vi "drone_havuz_uzaklık_uygulaması.vi"() -> ()   [LabVIEW 2018]
doc: "This example opens two VISA resources and configures one COM port to perform a write operation and the other COM port to perform a read operation. This VI will wait until the specified number of bytes is received at the port or until a termination character is read.\n\nThis example allows you perform diagnostic tests on your ports. You can use this example to perform a wrap-back test. Both serial ports must have the same basic configuration parameters. You can connect two of the ports using a null modem cable, which effectively connects one port's RX lines to the other port's TX lines. If you use a straight-through cable, one port's RX lines will be connected to the other port's RX lines, and you cannot communicate between the two ports."
uses:
  D:/Program Files (x86)/National Instruments/LabVIEW 2018/examples/Instrument IO/Serial/support/Serial - Settings.ctl
  <vilib>/Instr/_visa.llb/VISA Configure Serial Port (Instr).vi
panel:
  out "MESAFE GÖSTERGESİ":dbl(knob) scale=0.0..100.0
  out "Araç havuza çok uzak":bool
  out "Araç havuza uzak":bool
  out "Araç havuza yakın":bool
  in  "Termination Character":u8=10 format="%.0x"
  in  "End Write on Termination Character?":bool=TRUE
  in  "End Read on Termination Character?":bool=TRUE
  in  "Write String":string="*IDN?"
  in  "Serial Settings (read)":T1={"baud rate"=9600, "data bits"=8, "parity"=enum."None", "stop bits"=10, "flow control"=0} {"flow control" items=["None"=0, "XON/XOFF"=1, "RTS/CTS"=2, "DTR/DSR"=4]; "stop bits" items=["1.0"=10, "1.5"=15, "2.0"=20]; "data bits" min=5 max=8 step=1; "baud rate" items=["75"=75, "110"=110, "134"=134, "150"=150, "300"=300, "600"=600, "1200"=1200, "1800"=1800, "2400"=2400, "4800"=4800, "7200"=7200, "9600"=9600, "14400"=14400, "19200"=19200, "28800"=28800, "38400"=38400, "56000"=56000, "57600"=57600, "115200"=115200, "128000"=128000, "230400"=230400]}
  in  "Serial Settings (write)":T1={"baud rate"=9600, "data bits"=8, "parity"=enum."None", "stop bits"=10, "flow control"=0} {"flow control" items=["None"=0, "XON/XOFF"=1, "RTS/CTS"=2, "DTR/DSR"=4]; "stop bits" items=["1.0"=10, "1.5"=15, "2.0"=20]; "data bits" min=5 max=8 step=1; "baud rate" items=["75"=75, "110"=110, "134"=134, "150"=150, "300"=300, "600"=600, "1200"=1200, "1800"=1800, "2400"=2400, "4800"=4800, "7200"=7200, "9600"=9600, "14400"=14400, "19200"=19200, "28800"=28800, "38400"=38400, "56000"=56000, "57600"=57600, "115200"=115200, "128000"=128000, "230400"=230400]}
  out "bytes read":u32
  out "Read String":string
  in  "VISA Resource (read)":refnum<visa-resource-name>="COM2"
  out "bytes written":u32
  in  "VISA Resource (write)":refnum<visa-resource-name>="COM1"
  # "0xA is equivalent to a '\\n' character, which is a line feed."
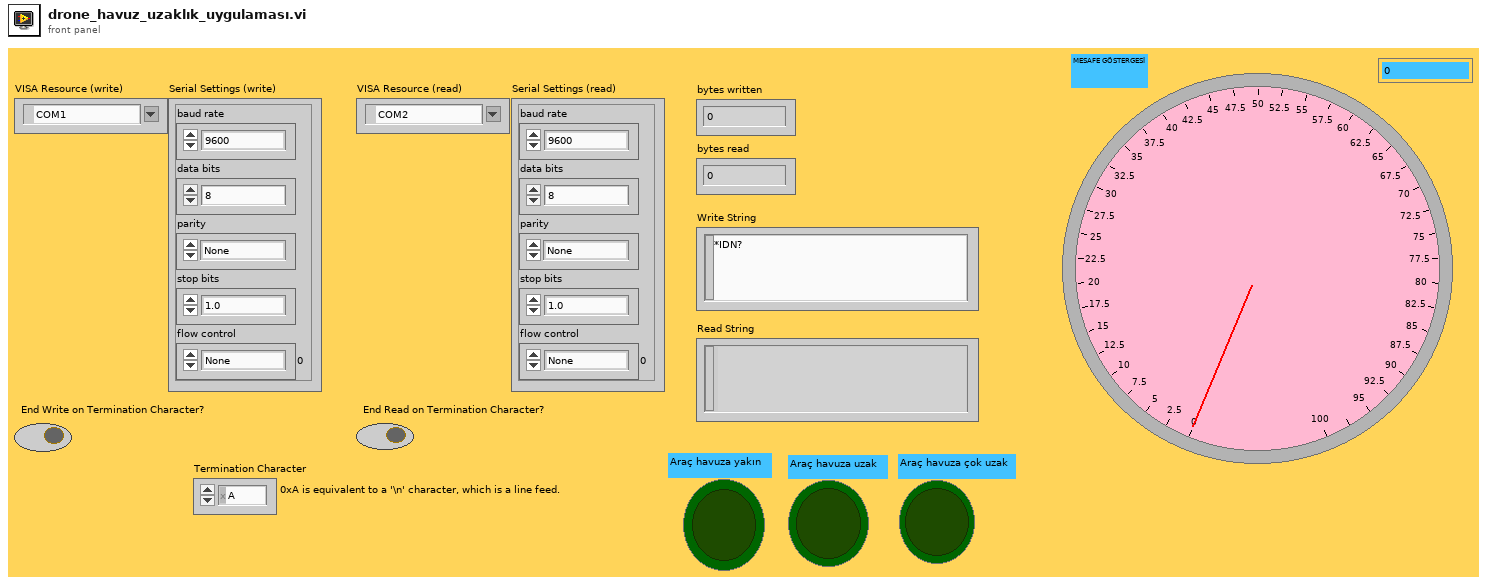
[diagram p1: front panel]
types:
  T1 = typedef "Serial - Settings.ctl" = cluster{"baud rate":u32, "data bits":u16, "parity":enum16{"None", "Odd", "Even", "Mark", "Space"}, "stop bits":u16, "flow control":u16}
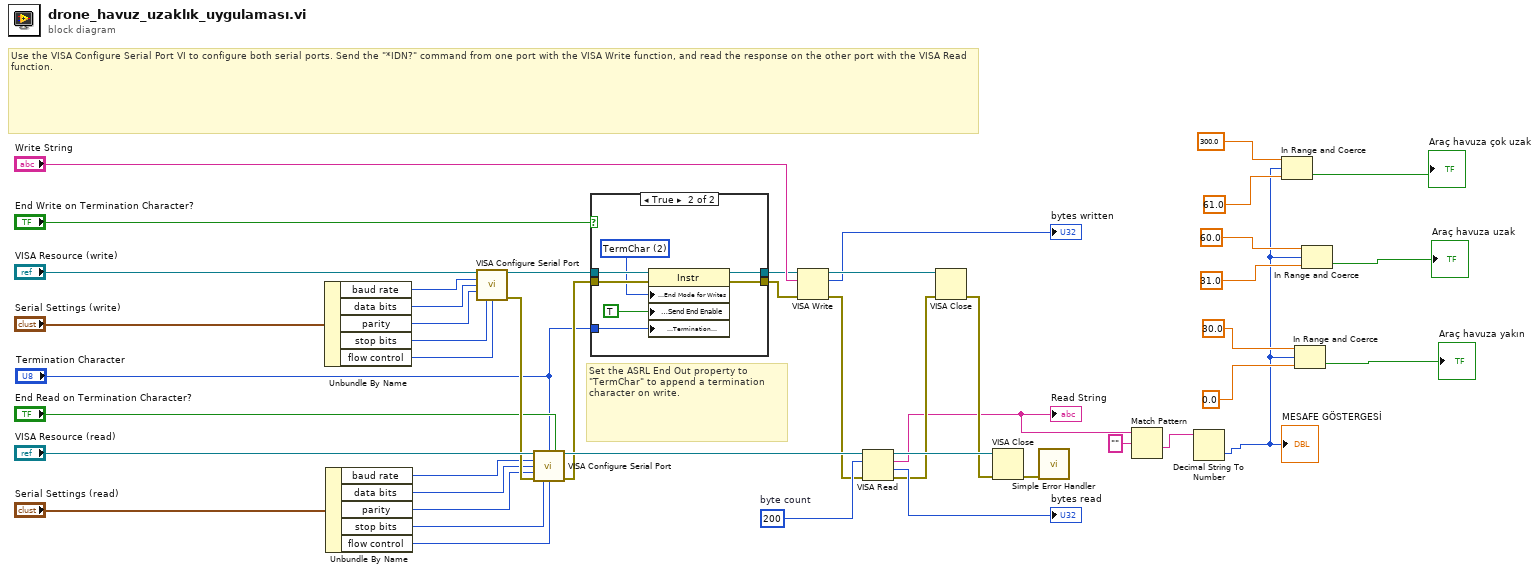
[diagram p0: block diagram]
diagram:
  w41 = u32 200  # byte count
  # "Set the ASRL End Out property to \"TermChar\" to append a termination character on write."
  # "Use the VISA Configure Serial Port VI to configure both serial ports. Send the \"*IDN?\" command from one port with the VISA Write function, and read the response on the other port with the VISA Read function."
  n1 = Unbundle By Name("Serial Settings (write)") -> ("baud rate"=w32:u32, "data bits"=w31:u16, "parity"=w30:enum16{"None", "Odd", "Even", "Mark", "Space"}, "stop bits"=w29:u16, "flow control"=w28:u16)
  n2 = Unbundle By Name("Serial Settings (read)") -> ("baud rate"=w26:u32, "data bits"=w25:u16, "parity"=w24:enum16{"None", "Odd", "Even", "Mark", "Space"}, "stop bits"=w23:u16, "flow control"=w22:u16)
  n3 = call-poly "VISA Configure Serial Port"("VISA resource name"="VISA Resource (write)", "baud rate (9600)"=w32, "data bits (8)"=w31, "parity (0:none)"=w30, "stop bits (10: 1 bit)"=w29, "flow control (0:none)"=w28) -> ("VISA resource name out"=w19:refnum<visa-resource-name>, "error out"=w38:errorcluster)  [unwired: 3 in, 5 out]
  n4 = call-poly "VISA Configure Serial Port"("VISA resource name"="VISA Resource (read)", "termination char\n(0xA = '\\n' = LF)"="Termination Character", "Enable Termination\nChar (T)"="End Read on Termination Character?", "baud rate (9600)"=w26, "data bits (8)"=w25, "parity (0:none)"=w24, "error in (no error)"=w38, "stop bits (10: 1 bit)"=w23, "flow control (0:none)"=w22) -> ("VISA resource name out"=w44:refnum<visa-resource-name>, "error out"=w17:errorcluster)  [unwired: 1 in, 4 out]
  n5 = case shown="True" "End Write on Termination Character?" {
    tunnel: w19 -> [w47 w55]
    tunnel: w17 -> [w48 w54]
    tunnel: [w47 w53] -> w18
    tunnel: [w48 w52] -> w16
    tunnel: "Termination Character" -> [_ w50]
    frame False {
    }
    frame True {
      w51 = u16 2 items=["None", "LastBit", "TermChar", "Break"] ("Serial Settings:Serial End Mode for Writes")
      n6 = property class="Instr"(reference=w55, error in=w54, "Serial Settings:End Mode for Writes"=w51, "Message Based Settings:Send End Enable"=TRUE, "Message Based Settings:Termination Character"=w50) -> (reference out=w53:refnum<visa-resource-name>, error out=w52:errorcluster)
    }
  }
  n7 = VISA Write(VISA resource name=w18, write buffer="Write String", error in (no error)=w16) -> (VISA resource name out=w45:refnum<visa-resource-name>, return count=→"bytes written":u32, error out=w37:errorcluster)
  n8 = VISA Read(VISA resource name=w44, byte count=w41, error in (no error)=w37) -> (VISA resource name out=w43:refnum<visa-resource-name>, read buffer=w13:string, return count=→"bytes read":u32, error out=w36:errorcluster)
  "Read String" <- w13
  n9 = VISA Close(VISA resource name=w45, error in (no error)=w36) -> (error out=w35:errorcluster)
  n10 = VISA Close(VISA resource name=w43, error in (no error)=w35) -> (error out=w34:errorcluster)
  n11 = call <vilib>:"Simple Error Handler.vi"("error in (no error)"=w34) -> ()  [unwired: 1 in, 8 out]
  n12 = Match Pattern(string=w13, regular expression="") -> (after substring=w11:string)  [unwired: 1 in, 3 out]
  n13 = Decimal String To Number(string=w11) -> (number=w1:i32)  [unwired: 2 in, 1 out]
  "MESAFE GÖSTERGESİ" <- w1
  n14 = In Range and Coerce(upper limit=300.0, x=w1, lower limit=61.0) -> (In Range?=→"Araç havuza çok uzak":bool)  [unwired: 1 out]
  n15 = In Range and Coerce(upper limit=30.0, x=w1, lower limit=0.0) -> (In Range?=→"Araç havuza yakın":bool)  [unwired: 1 out]
  n16 = In Range and Coerce(upper limit=60.0, x=w1, lower limit=31.0) -> (In Range?=→"Araç havuza uzak":bool)  [unwired: 1 out]
